vi "Configure External Trigger Level.vi"(8 "error in (no error)":errorcluster, 10 "Level (V)":dbl, 11 "DG645 in":refnum<class "DG645.lvclass">) -> (0 "error out":errorcluster, 3 "DG645 out":refnum<class "DG645.lvclass">)   [LabVIEW 2018, in "DG645.lvlib" / "DG645.lvclass"]
uses:
  DG645.lvclass
  DG645.lvclass/DG645.ctl
  <instrlib>/Stanford Research DG645/Stanford Research DG645.lvlib
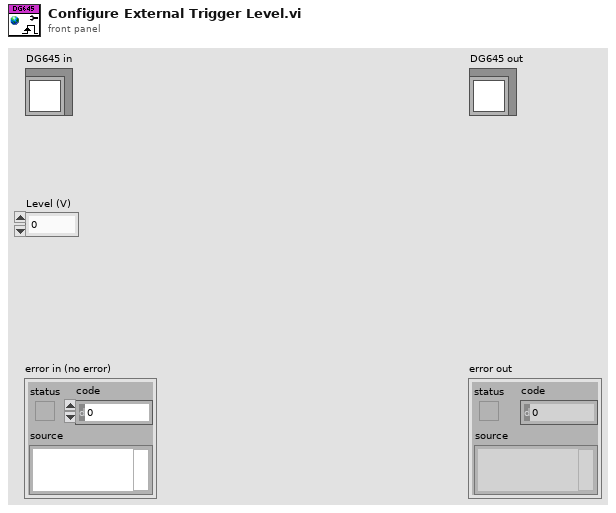
[diagram p1: front panel]
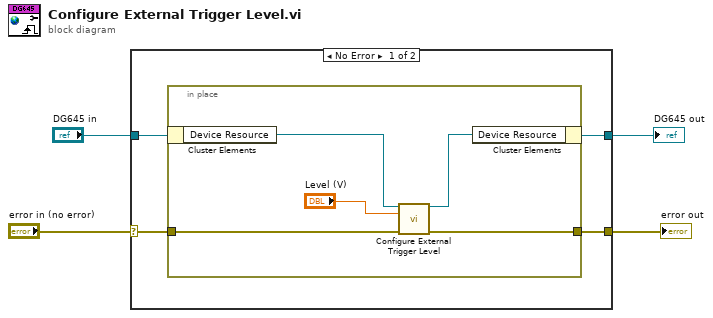
[diagram p0: block diagram]
diagram:
  n1 = case shown="No Error" "error in (no error)" {
    selector: "error in (no error)" -> [w7 w14]
    tunnel: "DG645 in" -> [w8 w15]
    tunnel: [w6 w14] -> w2
    tunnel: [w5 w15] -> w1
    frame No Error {
      n2 = in-place {
        in-place-border: w7 -> [w13]
        in-place-border: [w12] -> w6
        n3 = in-place-cluster #1(w8) -> ("Device Resource"=w11:refnum<visa-resource-name>)
        n4 = call <instrlib>:"Configure External Trigger Level.vi"("VISA resource name"=w11, "External Trigger Level (1 V)"="Level (V)", "error in (no error)"=w13) -> ("VISA resource name out"=w10:refnum<visa-resource-name>, "error out"=w12:errorcluster)  [unwired: 11 in]
        n5 = in-place-cluster #1("Device Resource"=w10) -> (w5:refnum<class "DG645.lvclass">)
      }
    }
    frame Error {
    }
  }
  "error out" <- w2
  "DG645 out" <- w1
